vi "Remove Previous Configurations by ID.vi"(8 "error in (no error)":errorcluster, 10 "Imported IDs":u16[](array[numeric]), 11 "Node In":u64) -> (0 "error out":errorcluster, 3 "Node Out":T1 format="%.0x")   [LabVIEW 2019, in "Diagnostics Addon System Explorer.lvlib"]
uses:
  Diagnostics Addon System Explorer.lvlib
  <vilib>/NI VeriStand/Custom Device API/Custom Device Item Ref.ctl
  <vilib>/NI VeriStand/Custom Device API/Custom Device API.lvlib
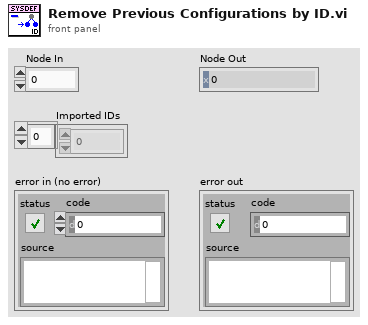
[diagram p1: front panel]
types:
  T1 = typedef "Custom Device API.lvlib/Custom Device Item Ref.ctl" = u64
  T2 = typedef "Custom Device API.lvlib/Custom Device Item Info.ctl" = cluster{"Name":string, "Is Channel":bool, "GUID":string, "Is Waveform":bool}
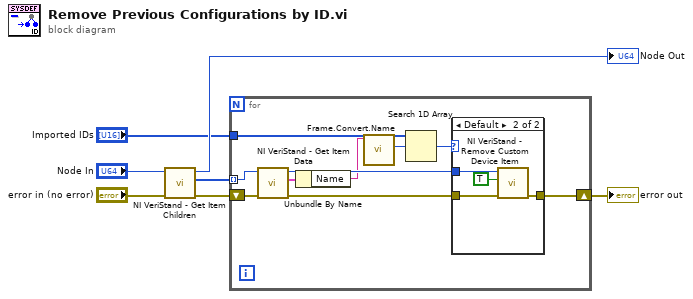
[diagram p0: block diagram]
diagram:
  n1 = call <vilib>:"NI VeriStand - Get Item Children.vi"("error in (no error)"="error in (no error)", "Item Ref in"="Node In") -> ("error out"=w1:errorcluster, "Child Refs"=w2:T1[], "Item Ref out"=→"Node Out":T1)  [unwired: 6 in, 1 out]
  n2 = for {
    shift-right: [w12] -> w6
    shift-left: w1 -> [w16]
    tunnel: w2 -> [w15] mode=indexing
    tunnel: "Imported IDs" -> [w14]
    n3 = call <vilib>:"NI VeriStand - Get Item Data.vi"("error in (no error)"=w16, "Item Ref in"=w15) -> ("error out"=w13:errorcluster, "Item Info"=w17:T2, "Item Ref out"=w11:T1)  [unwired: 7 out]
    n4 = Unbundle By Name(w17) -> ("Name"=w9:string)
    n5 = call "Frame.Convert.Name.vi"("VS Frame Name"=w9) -> ("ID"=w8:u16)  [unwired: 9 in, 1 out]
    n6 = Search 1D Array(1D array=w14, element=w8) -> (index of element=w10:i32)  [unwired: 1 in]
    n7 = case shown="Default" w10 {
      tunnel: w13 -> [w18 w22]
      tunnel: [w18 w21] -> w12
      tunnel: w11 -> [_ w20]
      frame -1 {
      }
      frame Default {
        n8 = call <vilib>:"NI VeriStand - Remove Custom Device Item.vi"("error in (no error)"=w22, "Force Delete (F)"=TRUE, "Item Ref in"=w20) -> ("error out"=w21:errorcluster)  [unwired: 7 in, 1 out]
      }
    }
  }
  "error out" <- w6
